vi "Excel Handle Headers for Printable.vi"(0 "CellsRefIn":refnum<k7>, 5 "HeaderInfo":string[](array[string]), 9 "IndexesPageStart":i32[](array[numeric]), 11 "ErrorIn":errorcluster) -> (4 "RefCellsOut":refnum<k7>, 15 "ErrorOut":errorcluster)   [LabVIEW 2013]
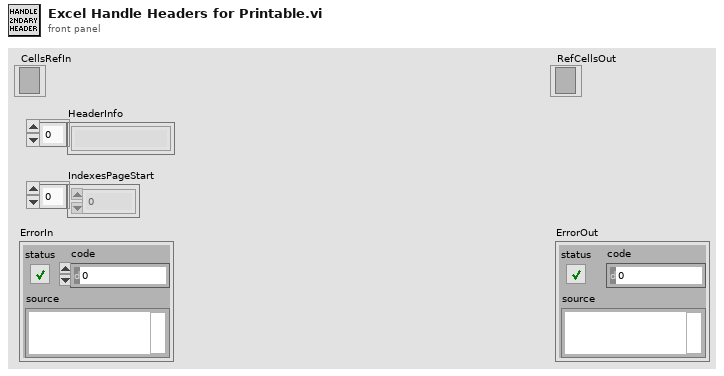
[diagram p1: front panel]
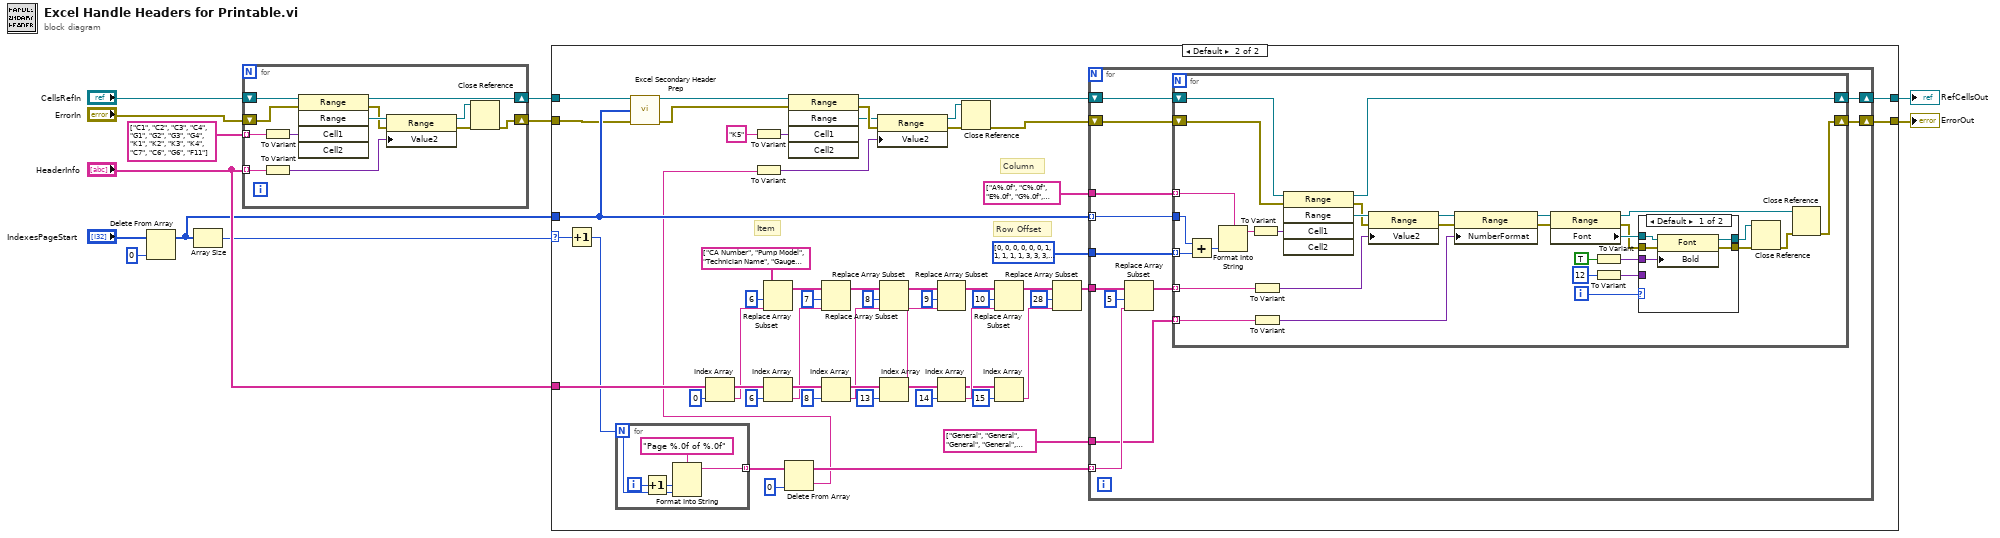
[diagram p0: block diagram]
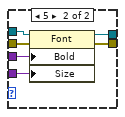
[diagram p3: hidden frame]
diagram:
  n1 = Delete From Array(array="IndexesPageStart", index=0) -> (array with subset deleted=w9:i32[])  [unwired: 1 in, 1 out]
  n2 = Array Size(array=w9) -> (size(s)=w2:i32)
  n3 = for {
    shift-right: [w19] -> w6
    shift-left: "ErrorIn" -> [w24]
    shift-right: [w18] -> w7
    shift-left: "CellsRefIn" -> [w17]
    tunnel: "HeaderInfo" -> [w16] mode=indexing
    tunnel: string[] ["C1", "C2", "C3", "C4", "G1", "G2", "G3", "G4", "K1", "K2", "K3", "K4", "C7", "C6", "G6", "F11"] -> [w15] mode=indexing
    n4 = To Variant(anything=w15) -> (Variant=w22:variant)
    n5 = To Variant(anything=w16) -> (Variant=w20:variant)
    n6 = invoke class="Range" method="Range"(reference=w17, error in=w24, "Cell1"=w22) -> (reference out=w18:refnum<k7>, error out=w21:errorcluster, "Range"=w23:refnum<k7>)  [unwired: 2 in, 2 out]
    n7 = property class="Range"(reference=w23, error in=w21, "Value2"=w20) -> (reference out=w14:refnum<k7>, error out=w13:errorcluster)
    n8 = Close Reference(reference=w14, error in (no error)=w13) -> (error out=w19:errorcluster)
  }
  n9 = case shown="Default" w2 {
    selector: w2 -> [_ w52]
    tunnel: "HeaderInfo" -> [_ w69]
    tunnel: w9 -> [_ w48]
    tunnel: w7 -> [w26 w47]
    tunnel: w6 -> [w25 w46]
    tunnel: [w26 w45] -> w3
    tunnel: [w25 w44] -> w1
    frame 0 {
    }
    frame Default {
      # "Row Offset"
      # "Column"
      # "Item"
      n10 = Increment(x=w52) -> (x+1=w51:i32)
      n11 = for {
        N: w51 -> [w135]
        tunnel: [w132] -> w42 mode=indexing
        i -> [w134]
        n12 = Increment(x=w134) -> (x+1=w133:i32)
        n13 = Format Into String(format string="Page %.0f of %.0f", w133, w135) -> (resulting string=w132:string)  [unwired: 2 in, 1 out]
      }
      n14 = call "Excel Secondary Header Prep.vi"("RefCellsIn"=w47, "[IndexPageStarts]"=w48, "ErrorIn"=w46) -> ("RefCellsOut"=w32:refnum<k7>, "ErrorOut"=w33:errorcluster)  [unwired: 11 in]
      n15 = Index Array(array=w69, index=0) -> (element=w65:string)
      n16 = To Variant(anything="K5") -> (Variant=w35:variant)
      n17 = Replace Array Subset(array=string[] ["CA Number", "Pump Model", "Technician Name", "Gauge Number", "Calibration Due Date", "***Place Holder***", "***Place Holder***", "***Place Holder***", "***Place Holder***", "***Place Holder***", "***Place Holder***", "Serial Number", "Voltage", "Pressure", "Flow", "Cont. Current", "Pump Current", "Speed", "Efficiency", "Fuel Temp", "Command", "Step", "Date", "'---", "(Volts)", "(kPa)", "(LPH)", "(Amps)", "***Placeholder***", "(RPM)", "(Percent)", "(Celsius)", "'---", "'---", "'---"], new element=w65, index=6) -> (w76:string[])
      n18 = Index Array(array=w69, index=6) -> (element=w66:string)
      n19 = Delete From Array(array=w42, index=0) -> (deleted portion=w29:string, array with subset deleted=w40:string[])  [unwired: 1 in]
      n20 = To Variant(anything=w29) -> (Variant=w37:variant)
      n21 = invoke class="Range" method="Range"(reference=w32, error in=w33, "Cell1"=w35) -> (reference out=w31:refnum<k7>, error out=w36:errorcluster, "Range"=w34:refnum<k7>)  [unwired: 2 in, 2 out]
      n22 = Replace Array Subset(array=w76, new element=w66, index=7) -> (w75:string[])
      n23 = Index Array(array=w69, index=8) -> (element=w67:string)
      n24 = property class="Range"(reference=w34, error in=w36, "Value2"=w37) -> (reference out=w38:refnum<k7>, error out=w39:errorcluster)
      n25 = Replace Array Subset(array=w75, new element=w67, index=8) -> (w74:string[])
      n26 = Index Array(array=w69, index=13) -> (element=w68:string)
      n27 = Replace Array Subset(array=w74, new element=w68, index=9) -> (w73:string[])
      n28 = Index Array(array=w69, index=14) -> (element=w70:string)
      n29 = Close Reference(reference=w38, error in (no error)=w39) -> (error out=w30:errorcluster)
      n30 = Replace Array Subset(array=w73, new element=w70, index=10) -> (w72:string[])
      n31 = Index Array(array=w69, index=15) -> (element=w71:string)
      n32 = Replace Array Subset(array=w72, new element=w71, index=28) -> (w50:string[])
      n33 = for {
        tunnel: w50 -> [w89]
        tunnel: w40 -> [w88] mode=indexing
        tunnel: i32[] [0, 0, 0, 0, 0, 0, 1, 1, 1, 1, 1, 3, 3, 3, 3, 3, 3, 3, 3, 3, 3, 3, 3, 4, 4, 4, 4, 4, 4, 4, 4, 4, 4, 4, 4] -> [w85]
        tunnel: string[] ["A%.0f", "C%.0f", "E%.0f", "G%.0f", "I%.0f", "K%.0f", "A%.0f", "C%.0f", "E%.0f", "G%.0f", "I%.0f", "A%.0f", "B%.0f", "C%.0f", "D%.0f", "E%.0f", "F%.0f", "G%.0f", "H%.0f", "I%.0f", "J%.0f", "K%.0f", "L%.0f", "A%.0f", "B%.0f", "C%.0f", "D%.0f", "E%.0f", "F%.0f", "G%.0f", "H%.0f", "I%.0f", "J%.0f", "K%.0f", "L%.0f"] -> [w86]
        tunnel: w48 -> [w83] mode=indexing
        shift-right: [w79] -> w45
        shift-left: w31 -> [w82]
        shift-right: [w80] -> w44
        shift-left: w30 -> [w81]
        tunnel: string[] ["General", "General", "General", "General", "General", "General", "General", "General", "General", "General", "m/d/yyyy", "General", "General", "General", "General", "General", "General", "General", "General", "General", "General", "General", "General", "General", "General", "General", "General", "General", "General", "General", "General", "General", "General", "General", "General"] -> [w78]
        n34 = Replace Array Subset(array=w89, new element=w88, index=5) -> (w84:string[])
        n35 = for {
          tunnel: w86 -> [w120] mode=indexing
          tunnel: w85 -> [w117] mode=indexing
          tunnel: w84 -> [w107] mode=indexing
          tunnel: w83 -> [w118]
          shift-right: [w113] -> w80
          shift-left: w81 -> [w116]
          shift-right: [w114] -> w79
          shift-left: w82 -> [w115]
          tunnel: w78 -> [w91] mode=indexing
          i -> [w96]
          n36 = Add(x=w118, y=w117) -> (x+y=w119:i32)
          n37 = Format Into String(format string=w120, w119) -> (resulting string=w108:string)  [unwired: 2 in, 1 out]
          n38 = To Variant(anything=w108) -> (Variant=w111:variant)
          n39 = To Variant(anything=w107) -> (Variant=w110:variant)
          n40 = To Variant(anything=w91) -> (Variant=w90:variant)
          n41 = invoke class="Range" method="Range"(reference=w115, error in=w116, "Cell1"=w111) -> (reference out=w114:refnum<k7>, error out=w109:errorcluster, "Range"=w112:refnum<k7>)  [unwired: 2 in, 2 out]
          n42 = property class="Range"(reference=w112, error in=w109, "Value2"=w110) -> (reference out=w95:refnum<k7>, error out=w94:errorcluster)
          n43 = property class="Range"(reference=w95, error in=w94, "NumberFormat"=w90) -> (reference out=w93:refnum<k7>, error out=w92:errorcluster)
          n44 = property class="Range"(reference=w93, error in=w92) -> (reference out=w99:refnum<k7>, error out=w103:errorcluster, "Font"=w106:refnum<k7>)
          n45 = To Variant(anything=TRUE) -> (Variant=w104:variant)
          n46 = To Variant(anything=12) -> (Variant=w97:variant)
          n47 = case shown="Default" w96 {
            tunnel: w106 -> [w125 w131]
            tunnel: w104 -> [w121 w130]
            tunnel: w103 -> [w124 w129]
            tunnel: [w123 w128] -> w102
            tunnel: [w122 w127] -> w101
            tunnel: w97 -> [_ w126]
            frame Default {
              n48 = property class="Font"(reference=w125, error in=w124, "Bold"=w121) -> (reference out=w122:refnum<k7>, error out=w123:errorcluster)
            }
            frame 5 {
              n49 = property class="Font"(reference=w131, error in=w129, "Bold"=w130, "Size"=w126) -> (reference out=w127:refnum<k7>, error out=w128:errorcluster)
            }
          }
          n50 = Close Reference(reference=w101, error in (no error)=w102) -> (error out=w100:errorcluster)
          n51 = Close Reference(reference=w99, error in (no error)=w100) -> (error out=w113:errorcluster)
        }
      }
    }
  }
  "RefCellsOut" <- w3
  "ErrorOut" <- w1
